vi "L31.vi"() -> ()   [LabVIEW 2014]
panel:
  in  "L31":dbl
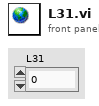
[diagram p1: front panel]
diagram:
